vi "Quasi-Harmonics.vi"(6 "Relative Freq":fxp<+,8,3>=1.0 format="%#_8g", 8 "1st partial":fxp<+,32,32>) -> (0 "Result Partial":fxp<+,32,32>)   [LabVIEW 2015]
doc: "Obtains a fractional (or integer) partial from a given frequency.\nThe relative frequency must be within [0, 7.96875].\n\nThe latency of this VI is 7 cycles."
uses:
  <vilib>/rvi/FXPMathLib/FxpMul/XNode/nifxpmath_Multiplier.xnode
  <vilib>/rvi/FXPMathLib/sim/FxpSim.dll
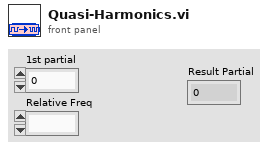
[diagram p1: front panel]
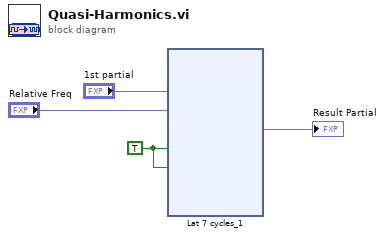
[diagram p0: block diagram]
diagram:
  w2 = TRUE ("input valid")
  n1 = xnode "Lat 7 cycles_1"("x"="1st partial", "y"="Relative Freq", "input valid"=w2, "ready for output (T)"=w2) -> ("x*y"=→"Result Partial":fxp<+,32,32>)  [unwired: 2 out]
